vi "test_vlp16_angle-data.vi"() -> ()   [LabVIEW 2019]
panel:
  out "XY Graph 4":cluster{sgl[], sgl[]}(graph)
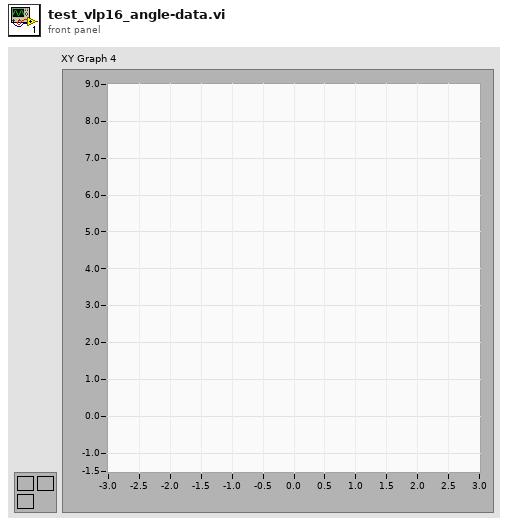
[diagram p1: front panel]
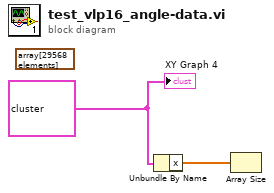
[diagram p0: block diagram]
diagram:
  w2 = cluster{"x":sgl[], "y":sgl[]} {"x"=array[29568 elements], "y"=array[29568 elements]} ("XY Graph")
  (unwired) cluster{"x":dbl, "y":dbl, "z":dbl}[] array[29568 elements] ("Array")
  n1 = Unbundle By Name(w2) -> ("x"=w1:sgl[])
  n2 = Array Size(array=w1) -> ()  [unwired: 1 out]
  "XY Graph 4" <- w2
